vi "Read.vi"(8 "error in (no error)":errorcluster, 11 "Data Class Array in":refnum<class "Data Class Array.lvclass">) -> (0 "error out":errorcluster, 2 "Data Class Array":refnum<class "Data Class.lvclass">[](array[class]), 3 "Data Class Array out":refnum<class "Data Class Array.lvclass">)   [LabVIEW 2020, in "Data.lvlib" / "Data Class Array.lvclass"]
doc: "Read Data Class Array."
uses:
  Data Class Array.lvclass
  Data Class/Data Class.lvclass
  Data Class Array.lvclass/Data Class Array.ctl
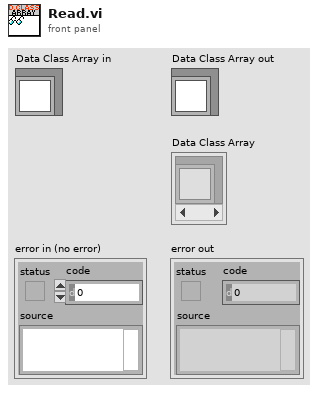
[diagram p1: front panel]
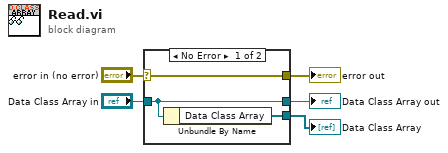
[diagram p0: block diagram]
diagram:
  n1 = case shown="No Error" "error in (no error)" {
    selector: "error in (no error)" -> [w8 w9]
    tunnel: [w8 w9] -> w4
    tunnel: [w7 w10] -> w2
    tunnel: "Data Class Array in" -> [w7 w10]
    tunnel: [w6 _] -> w1
    frame No Error {
      n2 = Unbundle By Name(w7) -> ("Data Class Array"=w6:refnum<class "Data Class.lvclass">[])
    }
    frame Error {
    }
  }
  "error out" <- w4
  "Data Class Array out" <- w2
  "Data Class Array" <- w1
